vi "SubVi-结果计算-主.vi"(0 "图像处理的结果字符串":string[](array[string])=["1324.431;855.439;56.642;56.854", "1344.162;933.603;49.796", "1313.304;289.485;163.904", "1180.462;813.487;874.380", "1179.184;649.118;875.954"], 5 "XY轴系数":string[][](array[string])=[["4.0064", "30578"], ["-4.0228", "9936.2"]], 7 "9点校正参数":string[][](table)=[["Null", "Null", "Null", "Null"], ["Null", "Null", "Null", "Null"], ["Null", "Null", "Null", "Null"], ["Null", "Null", "Null", "Null"], ["Null", "Null", "Null", "Null"]]) -> (3 "Distances X mm":dbl, 4 "结果数组":string[][](array[string]), 6 "结果数组":dbl[][](array[numeric]), 14 "Distances Y mm":dbl)   [LabVIEW 2015]
uses:
  <vilib>/vision/NI_Vision_Development_Module.lvlib
  <vilib>/Analysis/NI_AALPro.lvlib
panel:
  out "b2":dbl
  out "镜像值":cluster{"X":dbl, "Y":dbl}
  out "Y中心点":dbl
  out "X中心点":dbl
  out "K 镜像中心":dbl
  out "b1镜像中心":dbl
  out "添加的数组 2":cluster{"X":dbl, "Y":dbl}[](array[cluster])
  out "添加的数组":cluster{"X":sgl, "Y":sgl}[](array[cluster])
  out "元素":sgl
  out "L mm":dbl
  out "R mm":dbl
  out "9点校正后的数据":cluster{"X":dbl, "Y":dbl}[](array[cluster])
  # "第二次的不参与运算"
  # "第二次的不参与运算"
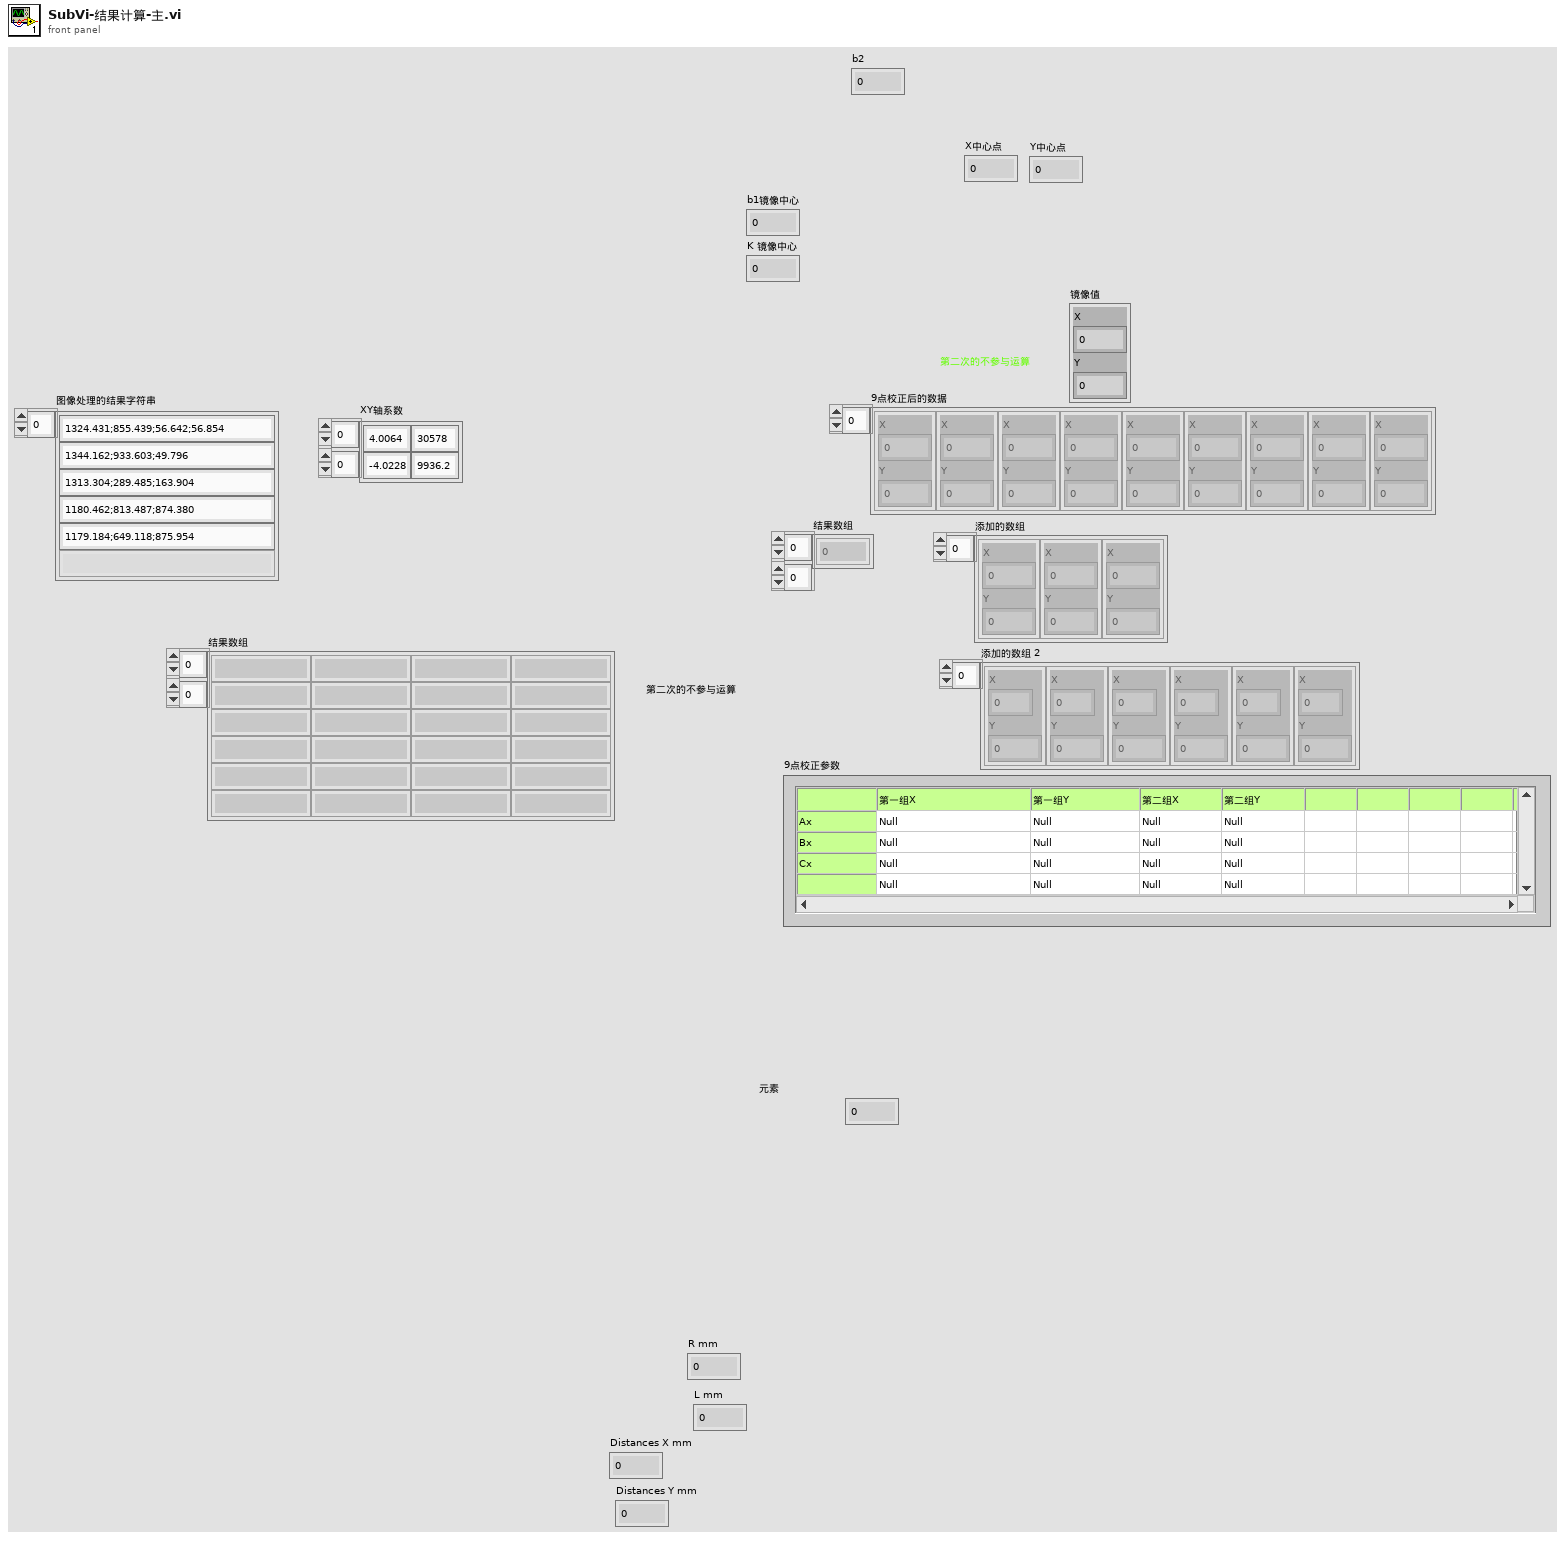
[diagram p1: front panel]
types:
  T1 = cluster{"Point 1":cluster{"X":sgl, "Y":sgl}, "Point 2":cluster{"X":sgl, "Y":sgl}}
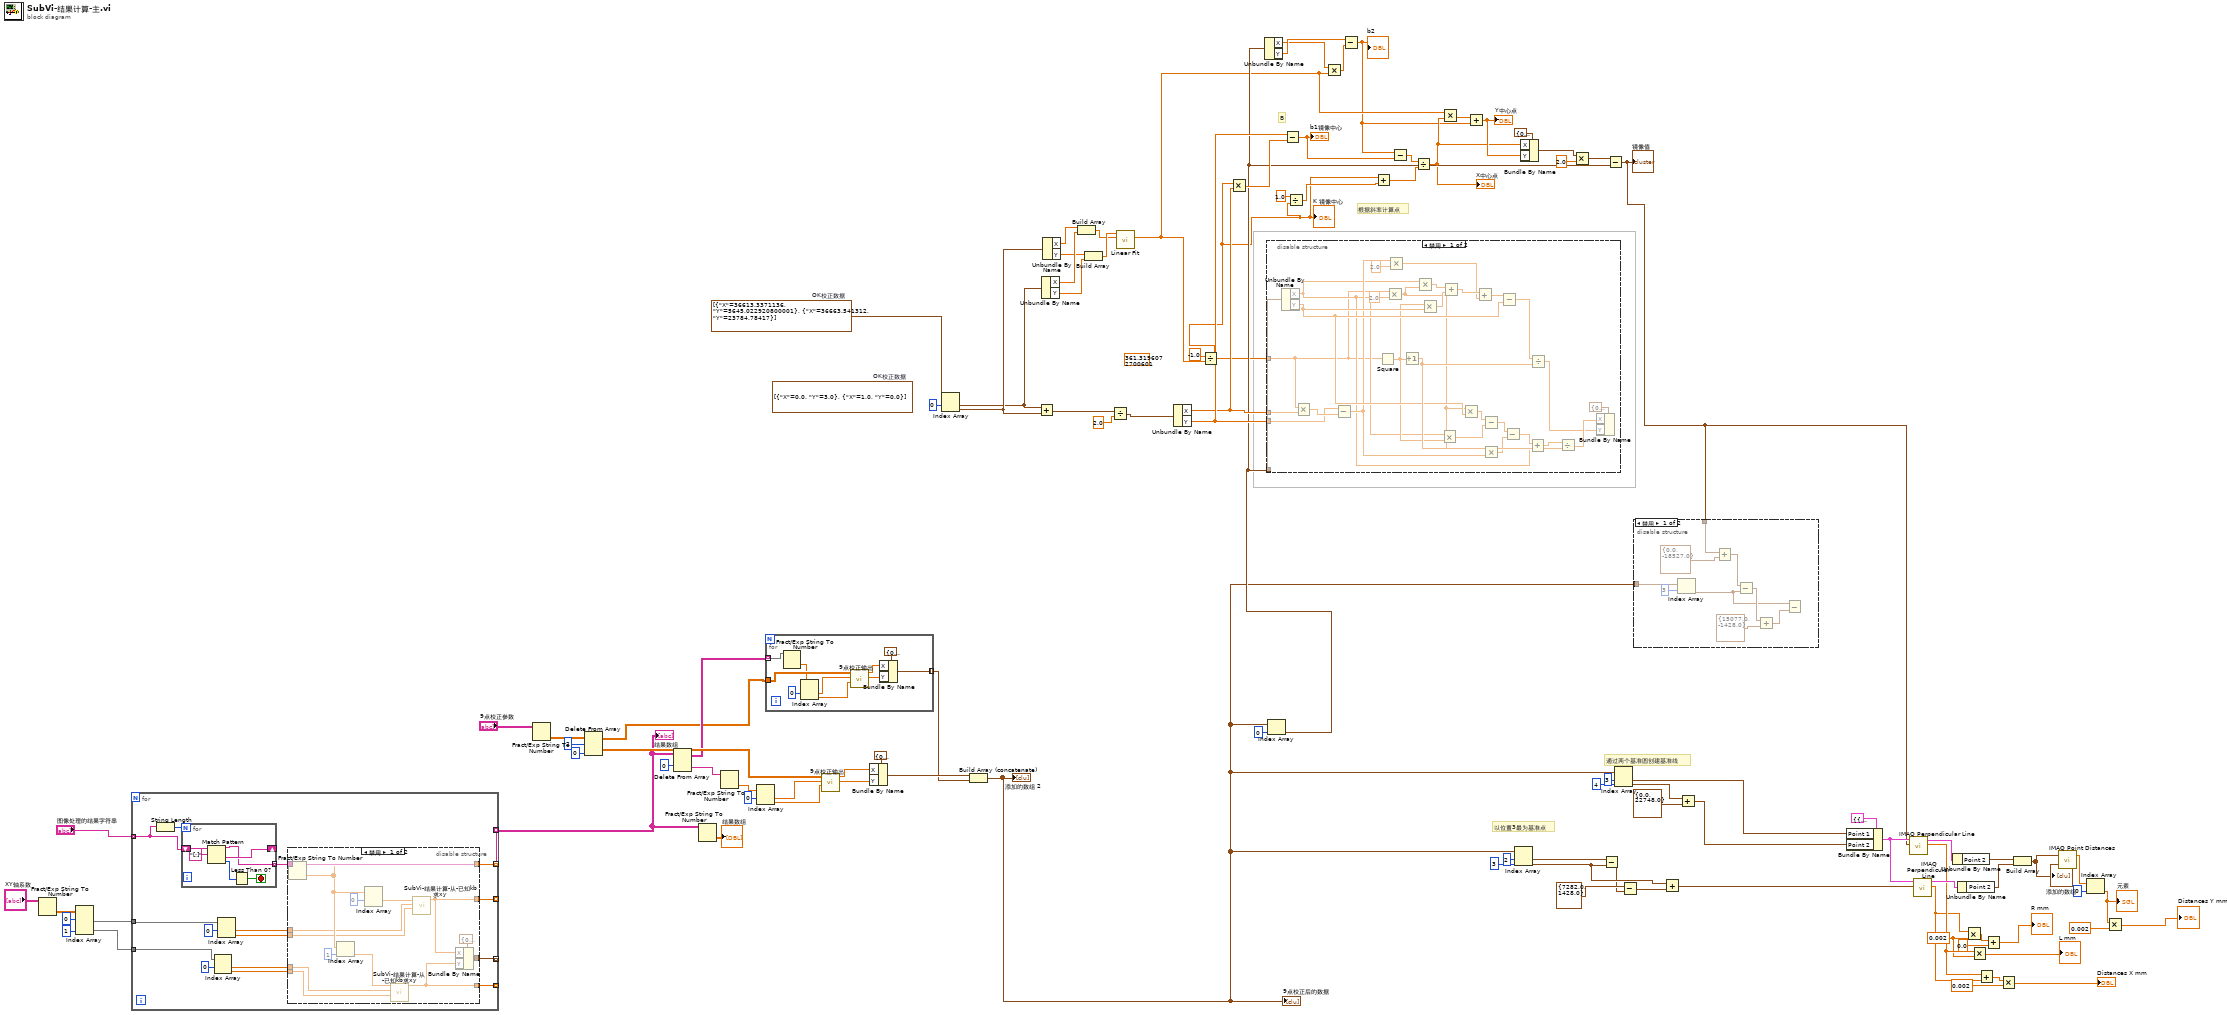
[diagram p0: block diagram]
diagram:
  w2 = cluster{"X":dbl, "Y":dbl}[] [{"X"=36613.3371136, "Y"=5645.022920800001}, {"X"=36663.541312, "Y"=23784.78417}]  # OK校正数据
  (unwired) 361.3196072700601 ("斜率")
  (unwired) cluster{"X":dbl, "Y":dbl}[] [{"X"=0.0, "Y"=3.0}, {"X"=1.0, "Y"=0.0}]  # OK校正数据
  w69 = 0.002 ("y")
  # "B"
  # "根据斜率计算点"
  # "以位置3最为基准点"
  # "通过两个基准圆创建基准线"
  n1 = Fract/Exp String To Number(string="XY轴系数") -> (number=w100:dbl[][])  [unwired: 3 in, 1 out]
  n2 = Index Array(array=w100, index (row) #1=0 ("索引 (行)"), index (row) #2=1 ("索引 (行)")) -> (element #1=w97:dbl[], element #2=w96:dbl[])  [unwired: 2 in]
  n3 = for {
    tunnel: "图像处理的结果字符串" -> [w117] mode=indexing
    tunnel: [w111] -> _ mode=indexing
    tunnel: w97 -> [w114]
    tunnel: w96 -> [w112]
    tunnel: [w106] -> _ mode=indexing
    tunnel: [w105] -> _ mode=indexing
    tunnel: [w104] -> _ mode=indexing
    tunnel: [w103] -> w40 mode=indexing
    n4 = String Length(string=w117) -> (length=w116:i32)
    n5 = for {
      N: w116 -> [_]
      shift-right: [w135] -> _
      shift-left: w117 -> [w137]
      tunnel: [w132] -> w103 mode=indexing
      stop <- w133 stop-if-true
      n6 = Match Pattern(string=w137, regular expression="[;]" ("正则表达式")) -> (before substring=w132:string, after substring=w135:string, offset past match=w134:i32)  [unwired: 1 in, 1 out]
      n7 = Less Than 0?(x=w134) -> (x < 0?=w133:bool)
    }
    n8 = Index Array(array=w112, index #1=0 ("索引")) -> (element #1=w108:dbl, element #2=w107:dbl)  [unwired: 1 in]
    n9 = Index Array(array=w114, index #1=0 ("索引")) -> (element #1=w110:dbl, element #2=w109:dbl)  [unwired: 1 in]
    n10 = disable-structure shown="禁用" {
      disable-tunnel: [w129 _] -> w111
      disable-tunnel: w110 -> [w127 _]
      disable-tunnel: w109 -> [w126 _]
      disable-tunnel: w108 -> [w124 _]
      disable-tunnel: w107 -> [w123 _]
      disable-tunnel: [w121 _] -> w106
      disable-tunnel: [w120 _] -> w105
      disable-tunnel: [w119 _] -> w104
      disable-tunnel: w103 -> [w118 _]
      frame Disabled {
        n11 = Fract/Exp String To Number(string=w118) -> (number=w129:dbl[])  [unwired: 3 in, 1 out]
        n12 = Index Array(array=w129, index=1 ("索引")) -> (element=w125:dbl)
        n13 = Index Array(array=w129, index #1=0 ("索引")) -> (element #1=w128:dbl)  [unwired: 1 in, 1 out]
        n14 = call "SubVi-结果计算-从-已知kb求xy.vi"("X-B"=w123, "X-K"=w124, "X value In"=w125) -> ("X value Out"=w120:dbl)  [unwired: 8 in]
        n15 = call "SubVi-结果计算-从-已知kb求xy.vi"("X-B"=w126, "X-K"=w127, "X value In"=w128) -> ("X value Out"=w121:dbl)  [unwired: 8 in]
        n16 = Bundle By Name(cluster=cluster{"X":dbl, "Y":dbl} {"X"=0.0, "Y"=0.0} ("输入簇"), "X"=w121, "Y"=w120) -> (w119:cluster{"X":dbl, "Y":dbl})
      }
      frame Enabled {
      }
    }
  }
  "结果数组" <- w40
  n17 = Fract/Exp String To Number(string="9点校正参数") -> (number=w56:dbl[][])  [unwired: 3 in, 1 out]
  n18 = Delete From Array(array=w56, length=2 ("长度"), index (col)=0 ("禁用的索引 (列)")) -> (deleted portion=w53:dbl[][], array with subset deleted=w43:dbl[][])  [unwired: 1 in]
  n19 = Delete From Array(array=w40, index (row)=0 ("索引 (行)")) -> (deleted portion=w52:string[], array with subset deleted=w44:string[][])  [unwired: 2 in]
  n20 = Fract/Exp String To Number(string=w40) -> (number=→"结果数组":dbl[][])  [unwired: 3 in, 1 out]
  n21 = Fract/Exp String To Number(string=w52) -> (number=w51:dbl[])  [unwired: 3 in, 1 out]
  n22 = Index Array(array=w51, index #1=0 ("索引")) -> (element #1=w49:dbl, element #2=w48:dbl)  [unwired: 1 in]
  n23 = for {
    tunnel: w44 -> [w140] mode=indexing
    tunnel: w43 -> [w141]
    tunnel: [w138] -> w41 mode=indexing
    n24 = Fract/Exp String To Number(string=w140) -> (number=w139:dbl[])  [unwired: 3 in, 1 out]
    n25 = Index Array(array=w139, index #1=0 ("索引")) -> (element #1=w143:dbl, element #2=w144:dbl)  [unwired: 1 in]
    n26 = call "9点校正输出.vi"("DY"=w144, "DX"=w143, "9点校正参数 输入"=w141) -> ("RY"=w147:dbl, "RX"=w146:dbl)  [unwired: 7 in]
    n27 = Bundle By Name(cluster=cluster{"X":dbl, "Y":dbl} {"X"=0.0, "Y"=0.0} ("输入簇"), "X"=w146, "Y"=w147) -> (w138:cluster{"X":dbl, "Y":dbl})
  }
  n28 = call "9点校正输出.vi"("DY"=w48, "DX"=w49, "9点校正参数 输入"=w53) -> ("RY"=w45:dbl, "RX"=w46:dbl)  [unwired: 7 in]
  n29 = Bundle By Name(cluster=cluster{"X":dbl, "Y":dbl} {"X"=0.0, "Y"=0.0} ("输入簇"), "X"=w46, "Y"=w45) -> (w42:cluster{"X":dbl, "Y":dbl})
  n30 = Index Array(array=w2, index #1=0 ("索引")) -> (element #1=w26:cluster{"X":dbl, "Y":dbl}, element #2=w27:cluster{"X":dbl, "Y":dbl})  [unwired: 1 in]
  n31 = Build Array (concatenate)(w42, w41) -> (w1:cluster{"X":dbl, "Y":dbl}[])
  "9点校正后的数据" <- w1
  "添加的数组 2" <- w1
  n32 = Add(x=w26, y=w27) -> (x+y=w36:cluster{"X":dbl, "Y":dbl})
  n33 = Unbundle By Name(w26) -> ("X"=w32:dbl, "Y"=w30:dbl)
  n34 = Unbundle By Name(w27) -> ("X"=w33:dbl, "Y"=w31:dbl)
  n35 = Build Array(w33, w32) -> (w28:dbl[])
  n36 = Build Array(w31, w30) -> (w29:dbl[])
  n37 = Divide(x=w36, y=2.0) -> (x/y=w34:cluster{"X":dbl, "Y":dbl})
  n38 = call <vilib>:"Linear Fit.vi"("Y"=w29, "X"=w28) -> ("slope"=w5:dbl)  [unwired: 9 in, 4 out]
  n39 = Unbundle By Name(w34) -> ("X"=w24:dbl, "Y"=w25:dbl)
  n40 = Divide(x=-1.0, y=w5) -> (x/y=w6:dbl)
  "K 镜像中心" <- w6
  n41 = Multiply(x=w6, y=w24) -> (x*y=w23:dbl)
  n42 = Index Array(array=w1, index=0 ("索引")) -> (element=w11:cluster{"X":dbl, "Y":dbl})
  n43 = Unbundle By Name(w11) -> ("X"=w9:dbl, "Y"=w10:dbl)
  n44 = disable-structure shown="禁用" {
    disable-tunnel: w11 -> [w151 _]
    disable-tunnel: w25 -> [w150 _]
    disable-tunnel: w24 -> [w149 _]
    disable-tunnel: w6 -> [w148 _]
    frame Disabled {
      n45 = Unbundle By Name(w151) -> ("X"=w156:dbl, "Y"=w165:dbl)
      n46 = Multiply(x=w148, y=w149) -> (x*y=w175:dbl)
      n47 = Subtract(x=w150, y=w175) -> (x-y=w159:dbl)
      n48 = Square(x=w148) -> (x^2=w163:dbl)
      n49 = Multiply(x=w148, y=2.0) -> (x*y=w160:dbl)
      n50 = Multiply(x=w159, y=2.0) -> (x*y=w168:dbl)
      n51 = Increment(x=w163) -> (x+1=w174:dbl)
      n52 = Multiply(x=w156, y=w160) -> (x*y=w172:dbl)
      n53 = Multiply(x=w163, y=w165) -> (x*y=w171:dbl)
      n54 = Multiply(x=w156, y=w163) -> (x*y=w162:dbl)
      n55 = Add(x=w172, y=w171) -> (x+y=w170:dbl)
      n56 = Multiply(x=w160, y=w165) -> (x*y=w164:dbl)
      n57 = Add(x=w170, y=w168) -> (x+y=w167:dbl)
      n58 = Subtract(x=w164, y=w162) -> (x-y=w161:dbl)
      n59 = Multiply(x=w160, y=w159) -> (x*y=w158:dbl)
      n60 = Subtract(x=w167, y=w165) -> (x-y=w166:dbl)
      n61 = Subtract(x=w161, y=w158) -> (x-y=w157:dbl)
      n62 = Add(x=w157, y=w156) -> (x+y=w152:dbl)
      n63 = Divide(x=w166, y=w174) -> (x/y=w153:dbl)
      n64 = Divide(x=w152, y=w174) -> (x/y=w154:dbl)
      n65 = Bundle By Name(cluster=cluster{"X":sgl, "Y":sgl} {"X"=0.0, "Y"=0.0} ("Point 1"), "X"=w154, "Y"=w153) -> ()  [unwired: 1 out]
    }
    frame Enabled {
    }
  }
  n66 = Subtract(x=w25, y=w23) -> (x-y=w7:dbl)
  "b1镜像中心" <- w7
  n67 = Divide(x=1.0, y=w6) -> (x/y=w19:dbl)
  n68 = Multiply(x=w9, y=w5) -> (x*y=w8:dbl)
  n69 = Subtract(x=w10, y=w8) -> (x-y=w3:dbl)
  "b2" <- w3
  n70 = Add(x=w6, y=w19) -> (x+y=w21:dbl)
  n71 = Subtract(x=w3, y=w7) -> (x-y=w22:dbl)
  n72 = Divide(x=w22, y=w21) -> (x/y=w4:dbl)
  "X中心点" <- w4
  n73 = Multiply(x=w5, y=w4) -> (x*y=w18:dbl)
  n74 = Add(x=w18, y=w3) -> (x+y=w16:dbl)
  "Y中心点" <- w16
  n75 = Index Array(array=w1, index #1=2 ("索引"), index #2=3 ("索引")) -> (element #1=w65:cluster{"X":dbl, "Y":dbl}, element #2=w63:cluster{"X":dbl, "Y":dbl})
  n76 = Bundle By Name(cluster=cluster{"X":sgl, "Y":sgl} {"X"=0.0, "Y"=0.0} ("Point 1"), "X"=w4, "Y"=w16) -> (w13:cluster{"X":sgl, "Y":sgl})
  n77 = Multiply(x=w13, y=2.0) -> (x*y=w14:cluster{"X":dbl, "Y":dbl})
  n78 = Subtract(x=w65, y=w63) -> (x-y=w61:cluster{"X":dbl, "Y":dbl})
  n79 = Subtract(x=w14, y=w11) -> (x-y=w12:cluster{"X":dbl, "Y":dbl})
  "镜像值" <- w12
  n80 = Index Array(array=w1, index #1=3 ("索引"), index #2=4 ("索引")) -> (element #1=w77:cluster{"X":dbl, "Y":dbl}, element #2=w80:cluster{"X":dbl, "Y":dbl})
  n81 = Subtract(x=cluster{"X":sgl, "Y":sgl} {"X"=7282.0, "Y"=1428.0} ("Point 1"), y=w61) -> (x-y=w64:cluster{"X":dbl, "Y":dbl})
  n82 = disable-structure shown="禁用" {
    disable-tunnel: w12 -> [w184 _]
    disable-tunnel: w1 -> [w176 _]
    frame Disabled {
      n83 = Index Array(array=w176, index=3 ("索引")) -> (element=w177:cluster{"X":dbl, "Y":dbl})
      n84 = Add(x=w184, y=cluster{"X":sgl, "Y":sgl} {"X"=0.0, "Y"=-18527.0} ("Point 1")) -> (x+y=w180:cluster{"X":dbl, "Y":dbl})
      n85 = Subtract(x=w180, y=w177) -> (x-y=w181:cluster{"X":dbl, "Y":dbl})
      n86 = Add(x=w181, y=cluster{"X":sgl, "Y":sgl} {"X"=15077.0, "Y"=-1428.0} ("Point 1")) -> (x+y=w179:cluster{"X":dbl, "Y":dbl})
      n87 = Subtract(x=w177, y=w179) -> ()  [unwired: 1 out]
    }
    frame Enabled {
    }
  }
  n88 = Add(x=w63, y=w64) -> (x+y=w66:cluster{"X":dbl, "Y":dbl})
  n89 = Add(x=w80, y=cluster{"X":sgl, "Y":sgl} {"X"=0.0, "Y"=22748.0} ("Point 1")) -> (x+y=w76:cluster{"X":dbl, "Y":dbl})
  n90 = Bundle By Name(cluster=T1 {"Point 1"={"X"=0.0, "Y"=0.0}, "Point 2"={"X"=0.0, "Y"=0.0}} ("Line"), "Point 1"=w77, "Point 2"=w76) -> (w92:T1)
  n91 = call "IMAQ Perpendicular Line"("Point"=w12, "Line"=w92) -> ("Distance"=w74:dbl, "Perpendicular Line"=w59:T1)  [unwired: 7 in, 1 out]
  n92 = call "IMAQ Perpendicular Line"("Point"=w66, "Line"=w92) -> ("Distance"=w68:dbl, "Perpendicular Line"=w91:T1)  [unwired: 7 in, 1 out]
  n93 = Unbundle By Name(w59) -> ("Point 2"=w90:cluster{"X":sgl, "Y":sgl})
  n94 = Unbundle By Name(w91) -> ("Point 2"=w89:cluster{"X":sgl, "Y":sgl})
  n95 = Multiply(x=w68, y=w69) -> (x*y=w72:dbl)
  n96 = Multiply(x=w74, y=w69) -> (x*y=→"L mm":dbl)
  n97 = Add(x=w74, y=w68) -> (x+y=w84:dbl)
  n98 = Add(x=w72, y=0.0) -> (x+y=→"R mm":dbl)
  n99 = Multiply(x=w84, y=0.002) -> (x*y=→"Distances X mm":dbl)
  n100 = Build Array(w90, w89) -> (w88:cluster{"X":sgl, "Y":sgl}[])
  "添加的数组" <- w88
  n101 = call "IMAQ Point Distances"("Points"=w88) -> ("Distances"=w87:sgl[])  [unwired: 4 in, 1 out]
  n102 = Index Array(array=w87, index=0 ("索引")) -> (element=w81:sgl)
  "元素" <- w81
  n103 = Multiply(x=w81, y=0.002) -> (x*y=→"Distances Y mm":dbl)
